vi "Python@File__Parameter.vi"(1 "ParamterIn":string) -> (0 "ParamterOut":string)   [LabVIEW 2020]
uses:
  MainFrame/Global.vi
panel:
  in  "FileName":string(combo)
  in  "Confirm":bool
  # "Python@File $PythonFile"
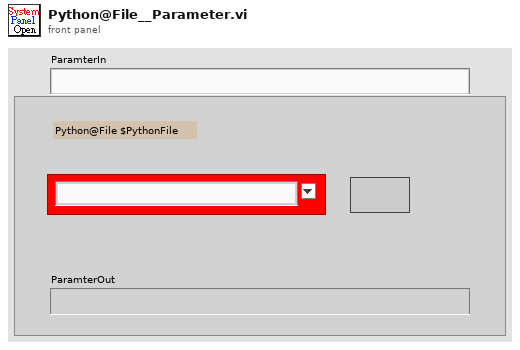
[diagram p1: front panel]
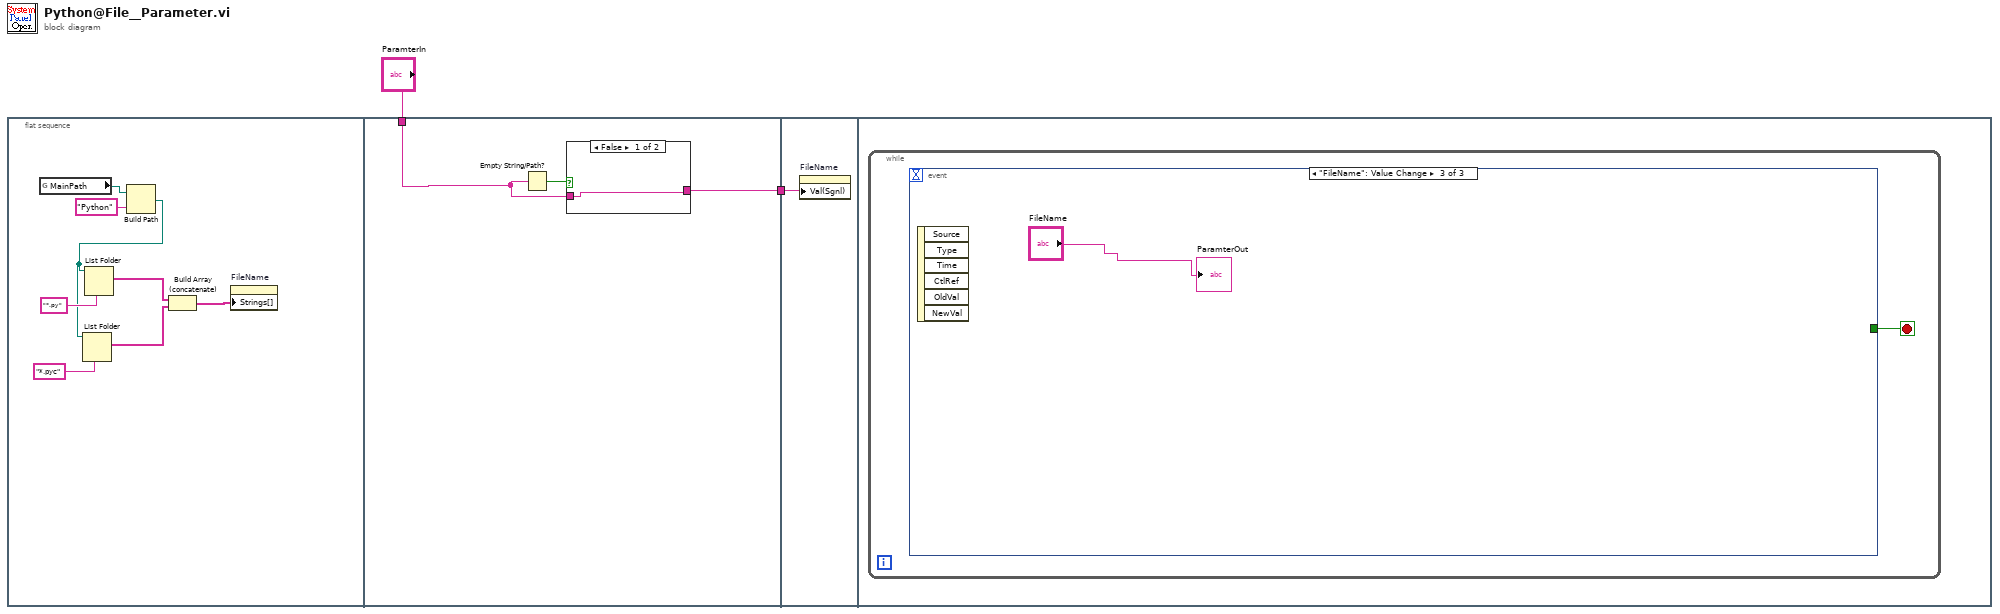
[diagram p0: block diagram]
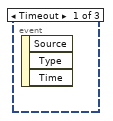
[diagram p3: hidden frame]
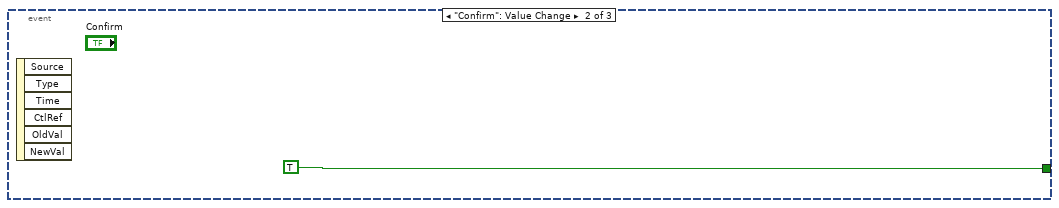
[diagram p4: hidden frame]
diagram:
  n1 = flat-sequence {
    tunnel: "ParamterIn" -> [w11]
    tunnel: [w12] -> w1
    tunnel: w1 -> [w16]
    frame #0 {
      n2 = global read "Global.vi" "MainPath"() -> (w9:path)
      n3 = Build Path(base path=w9, name or relative path="Python") -> (appended path=w6:path)
      n4 = List Folder(path=w6, pattern="*.pyc") -> (filenames=w4:string[])  [unwired: 2 in, 3 out]
      n5 = List Folder(path=w6, pattern="*.py") -> (filenames=w5:string[])  [unwired: 2 in, 3 out]
      n6 = Build Array (concatenate)(w5, w4) -> (w3:string[])
      n7 = property on="FileName" class="CmbBox"("Strings[]"=w3) -> ()  [unwired: 2 in, 2 out]
    }
    frame #1 {
      n8 = Empty String/Path?(string/path=w11) -> (empty?=w13:bool)
      n9 = case shown="False" w13 {
        tunnel: w11 -> [w14 w15]
        tunnel: [w14 w15] -> w12
        frame False {
        }
        frame True {
        }
      }
    }
    frame #2 {
      n10 = property on="FileName" class="CmbBox"("Val(Sgnl)"=w16) -> ()  [unwired: 2 in, 2 out]
    }
    frame #3 {
      n11 = while {
        stop <- w17 stop-if-true
        n12 = event shown="[2] \"FileName\": Value Change" {
          selector: _ -> [_ _ _]
          dyn-events: _ -> [_ _ _]
          timeout: _ -> [_ _ _]
          tunnel: [_ TRUE _] -> w17
          event Timeout {
            n13 = event-data() -> ()  [unwired: 1 in, 3 out]
          }
          event "Confirm": Value Change {
            n14 = event-data() -> ()  [unwired: 1 in, 6 out]
          }
          event "FileName": Value Change {
            n15 = event-data() -> ()  [unwired: 1 in, 6 out]
            "ParamterOut" <- "FileName"
          }
        }
      }
    }
  }
